vi "Joke Creator.vi"(10 "Name Two":string, 11 "Name One":string) -> (3 "Resulting Prompt":string)   [LabVIEW 2025, in "MCP Demo Application.lvlib"]
uses:
  MCP Demo Application.lvlib
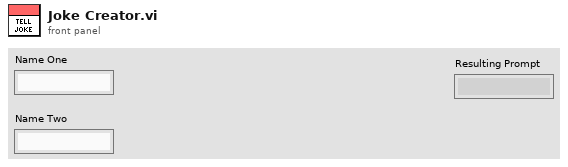
[diagram p1: front panel]
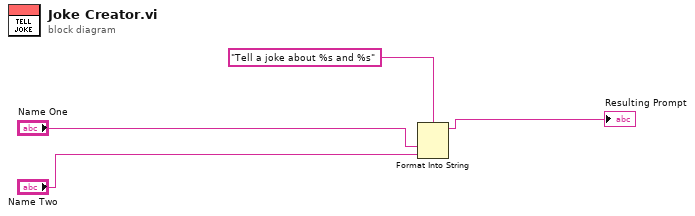
[diagram p0: block diagram]
diagram:
  n1 = Format Into String(format string="Tell a joke about %s and %s", "Name One", "Name Two") -> (resulting string=→"Resulting Prompt":string)  [unwired: 2 in, 1 out]
